vi "Undo.vi"(0 "reference in":refnum<class "PauseMusicCommand.lvclass">, 11 "Error In":errorcluster) -> (4 "reference out":refnum<class "PauseMusicCommand.lvclass">, 15 "Error Out":errorcluster)   [LabVIEW 2024, in "PauseMusicCommand.lvclass"]
doc: "Calls MediaPlayer and pauses music (opposite of play)."
uses:
  PauseMusicCommand.lvclass
  PauseMusicCommand.lvclass/PauseMusicCommand.ctl
  MediaPlayer_class/MediaPlayer.lvclass
panel:
  # "Connector Pane"
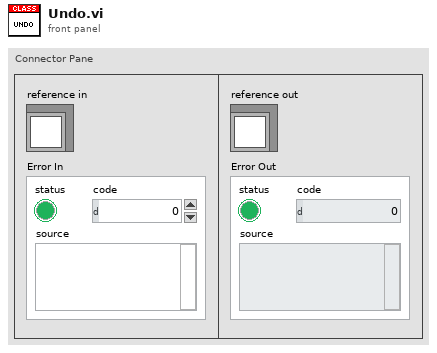
[diagram p1: front panel]
types:
  T1 = typedef "PauseMusicCommand.lvclass/ObjectAttributes.ctl" = cluster{"MediaPlayerRef":refnum<class "MediaPlayer.lvclass">}
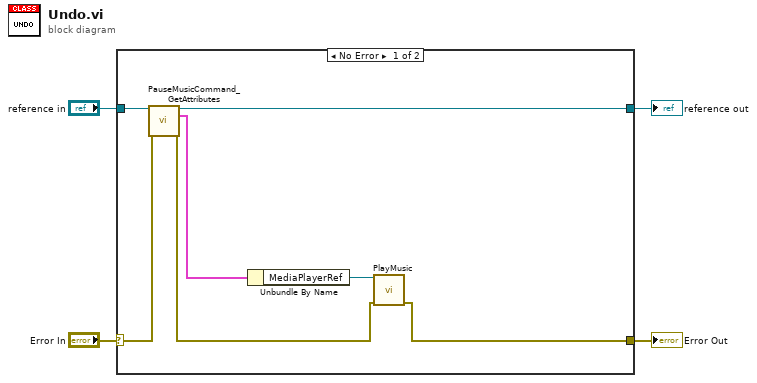
[diagram p0: block diagram]
diagram:
  n1 = case shown="No Error" "Error In" {
    selector: "Error In" -> [w11 w13]
    tunnel: [w5 w13] -> w3
    tunnel: [w8 w12] -> w1
    tunnel: "reference in" -> [w9 w12]
    frame No Error {
      n2 = call "PauseMusicCommand_GetAttributes.vi"("reference in"=w9, "Error In"=w11) -> ("reference out"=w8:refnum<class "PauseMusicCommand.lvclass">, "Data"=w10:T1, "Error Out"=w6:errorcluster)  [unwired: 10 in, 1 out]
      n3 = Unbundle By Name(w10) -> ("MediaPlayerRef"=w7:refnum<class "MediaPlayer.lvclass">)
      n4 = call-dynamic "PlayMusic.vi"("reference in"=w7, "Error In"=w6) -> ("Error Out"=w5:errorcluster)  [unwired: 12 in, 1 out]
    }
    frame Error {
    }
  }
  "Error Out" <- w3
  "reference out" <- w1
